vi "Process.vi"(8 "error in (no error)":errorcluster, 10 "Message in":refnum<class "Message.lvclass">, 11 "Architecture.lvlib:Thread.lvclass":refnum<class "Thread.lvclass">) -> (0 "error out":errorcluster, 1 "Stop?":bool, 3 "Architecture.lvlib:Thread.lvclass 2":refnum<class "Thread.lvclass">)   [LabVIEW 2012, in "Architecture.lvlib" / "Message.lvclass"]
uses:
  Message.lvclass
  Thread/Thread.lvclass
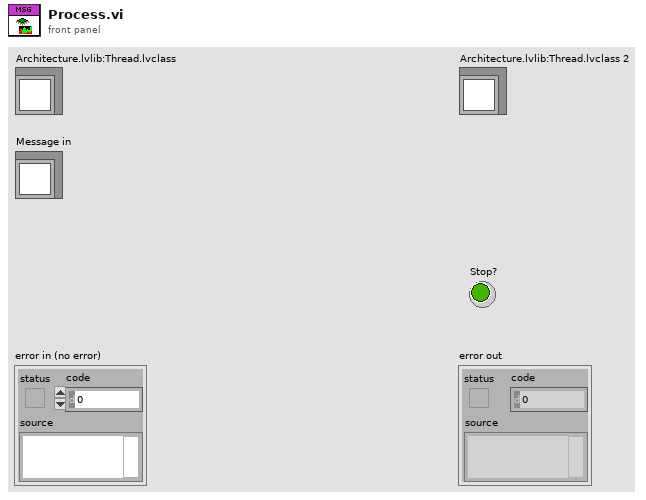
[diagram p1: front panel]
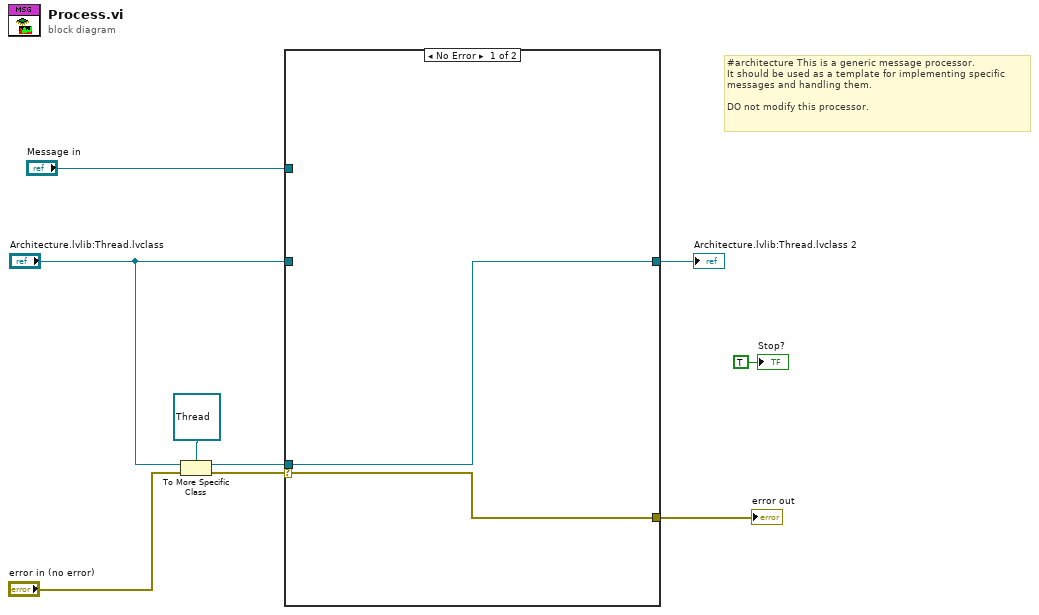
[diagram p0: block diagram]
diagram:
  # "#architecture This is a generic message processor.\nIt should be used as a template for implementing specific\nmessages and handling them.\n\nDO not modify this processor."
  n1 = To More Specific Class(target class=refnum<class "Thread.lvclass"> refnum, reference="Architecture.lvlib:Thread.lvclass", error in="error in (no error)") -> (specific class reference=w6:refnum<class "Thread.lvclass">, error out=w7:errorcluster)
  n2 = case shown="No Error" w7 {
    selector: w7 -> [w10 w12]
    tunnel: w6 -> [w11 _]
    tunnel: [w11 w13] -> w5
    tunnel: "Architecture.lvlib:Thread.lvclass" -> [_ w13]
    tunnel: [w10 w12] -> w2
    tunnel: "Message in" -> [_ _]
    frame No Error {
    }
    frame Error {
    }
  }
  "error out" <- w2
  "Architecture.lvlib:Thread.lvclass 2" <- w5
  "Stop?" <- TRUE ("Stop?")
